vi "get-long-term.vi"(2 "Ilims":cluster{"i(Pmax)":dbl, "i(Pmin)":dbl}, 3 "param":T1={"Srated"=25000.0, "eta [pu]"=0.98, "model"={"in-states"={"v1"=0.0, "v2"=0.0, "SoC"=0.0}, "output"={"V"=0.0, "Zeq"=0.0, "Eeq"=0.0}}} {"model"."output"."Eeq" format="%#.6g"; "model"."output"."Zeq" format="%#.6g"; "eta [pu]" format="%#_13g"}) -> (0 "Pmax":dbl, 1 "Pmin":dbl)   [LabVIEW 2021]
uses:
  General purpose/agent-variables.ctl
panel:
  out "Pmaxmaxs":dbl[](array[numeric])
  out "Pminmins":dbl[](array[numeric])
  in  "model-dt":u32=100
  in  "nr-of-timesteps":i32=9
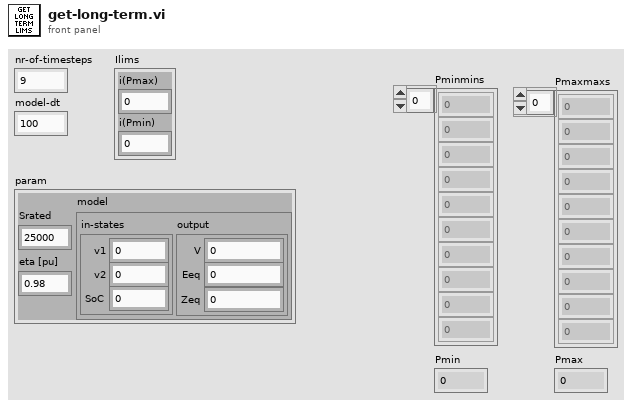
[diagram p1: front panel]
types:
  T1 = typedef "agent-variables.ctl" = cluster{"Srated":dbl, "eta [pu]":dbl, "model":cluster{"in-states":cluster{"v1":dbl, "v2":dbl, "SoC":dbl}, "output":cluster{"V":dbl, "Zeq":dbl, "Eeq":dbl}}}
  T2 = cluster{"in-states":cluster{"v1":dbl, "v2":dbl, "SoC":dbl}, "output":cluster{"V":dbl, "Zeq":dbl, "Eeq":dbl}}
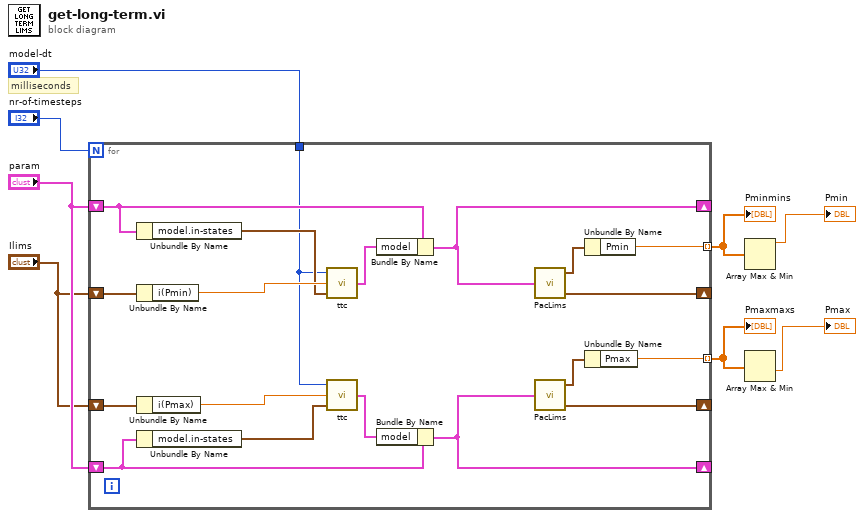
[diagram p0: block diagram]
diagram:
  # "milliseconds"
  n1 = for {
    N: "nr-of-timesteps" -> [_]
    tunnel: [w23] -> w8 mode=indexing
    tunnel: [w22] -> w7 mode=indexing
    shift-right: [w16] -> _
    shift-left: "param" -> [w18]
    shift-right: [w15] -> _
    shift-left: "param" -> [w17]
    tunnel: "model-dt" -> [w14]
    shift-right: [w9] -> _
    shift-left: "Ilims" -> [w12]
    shift-right: [w11] -> _
    shift-left: "Ilims" -> [w13]
    n2 = Unbundle By Name(w18) -> ("model.in-states"=w20:cluster{"v1":dbl, "v2":dbl, "SoC":dbl})
    n3 = Unbundle By Name(w13) -> ("i(Pmin)"=w26:dbl)
    n4 = Unbundle By Name(w12) -> ("i(Pmax)"=w10:dbl)
    n5 = Unbundle By Name(w17) -> ("model.in-states"=w27:cluster{"v1":dbl, "v2":dbl, "SoC":dbl})
    n6 = call "ttc.vi"("x[k-1]"=w20, "I"=w26, "Period"=w14) -> ("model"=w21:T2)  [unwired: 2 in]
    n7 = call "ttc.vi"("x[k-1]"=w27, "I"=w10, "Period"=w14) -> ("model"=w19:T2)  [unwired: 2 in]
    n8 = Bundle By Name(cluster=w18, "model"=w21) -> (w16:T1)
    n9 = Bundle By Name(cluster=w17, "model"=w19) -> (w15:T1)
    n10 = call "PacLims.vi"("param (in)"=w16) -> ("PacLims"=w25:cluster{"Pmax":dbl, "Pmin":dbl}, "Ilims"=w11:cluster{"i(Pmax)":dbl, "i(Pmin)":dbl})  [unwired: 1 out]
    n11 = call "PacLims.vi"("param (in)"=w15) -> ("PacLims"=w24:cluster{"Pmax":dbl, "Pmin":dbl}, "Ilims"=w9:cluster{"i(Pmax)":dbl, "i(Pmin)":dbl})  [unwired: 1 out]
    n12 = Unbundle By Name(w25) -> ("Pmin"=w23:dbl)
    n13 = Unbundle By Name(w24) -> ("Pmax"=w22:dbl)
  }
  "Pminmins" <- w8
  "Pmaxmaxs" <- w7
  n14 = Array Max & Min(array=w8) -> (max value=→"Pmin":dbl)  [unwired: 3 out]
  n15 = Array Max & Min(array=w7) -> (min value=→"Pmax":dbl)  [unwired: 3 out]
